vi "ReadPAQdata.vi"(4 "Tags":string[](array[string]), 6 "TableName":string, 8 "error in (no error)":errorcluster, 9 "Time-End":timestamp, 10 "Time-Start":timestamp, 11 "DBAL in":refnum<class "DBAL.lvclass">) -> (0 "error out":errorcluster, 2 "PAQ_section":T1, 3 "DBAL out":refnum<class "DBAL.lvclass">)   [LabVIEW 2020, in "Sgraph_lib_V1.lvlib" / "DBAL.lvclass"]
doc: "Andre Koelewijn,m 8 may 2021\n\nRead a number of PAQ TAGs from a specific time span from the database"
uses:
  DBAL.lvclass
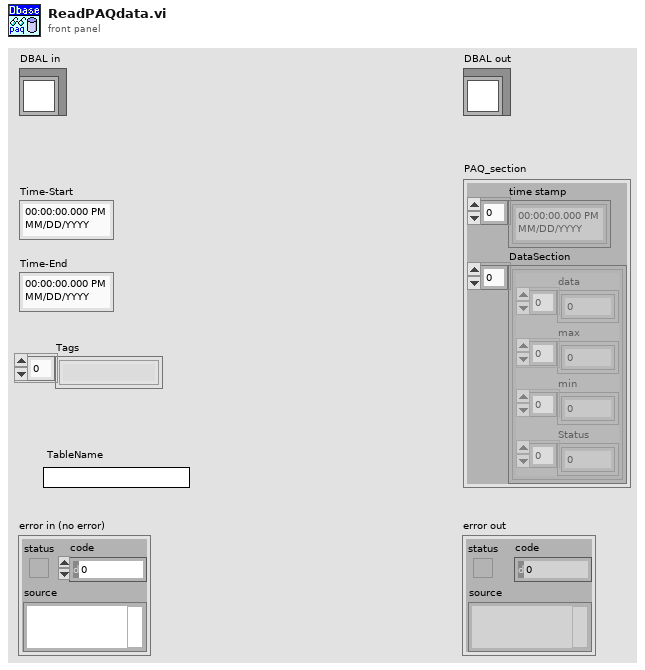
[diagram p1: front panel]
types:
  T1 = cluster{"time stamp":timestamp[], "DataSection":cluster{"data":dbl[], "max":dbl[], "min":dbl[], "Status":u32[]}[]}
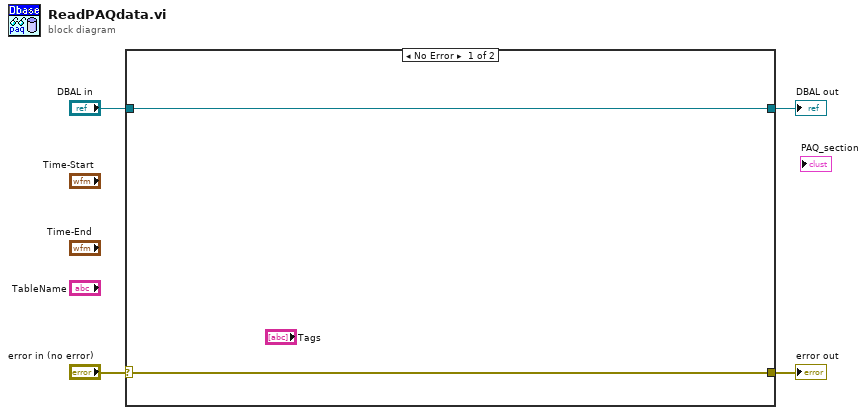
[diagram p0: block diagram]
diagram:
  n1 = case shown="No Error" "error in (no error)" {
    selector: "error in (no error)" -> [w5 w8]
    tunnel: [w5 w8] -> w3
    tunnel: [w6 w7] -> w1
    tunnel: "DBAL in" -> [w6 w7]
    frame No Error {
    }
    frame Error {
    }
  }
  "error out" <- w3
  "DBAL out" <- w1
